vi "ActionVIOnRecompile.vi"(8 "error in":errorcluster, 9 "Timeout (ms)":u32, 10 "Runtime Configurable Section Path":string, 11 "Device Item Ref in":T1 format="%.0x") -> (0 "error out":errorcluster)   [LabVIEW 2020]
uses:
  <vilib>/NI VeriStand/Custom Device API/Custom Device Item Ref.ctl
  <vilib>/NI VeriStand/Custom Device API/Custom Device Channel Type.ctl
  <vilib>/NI VeriStand/Custom Device API/Data Access Type.ctl
  <vilib>/NI VeriStand/Execution/CustomDevice/NI VeriStand - Send Custom Device Message (Byte Array).vi
  <vilib>/NI VeriStand/Custom Device API/Custom Device API.lvlib
  <vilib>/NI VeriStand/Execution/CustomDevice/NI_VS Custom Device ExecutionAPI.lvlib
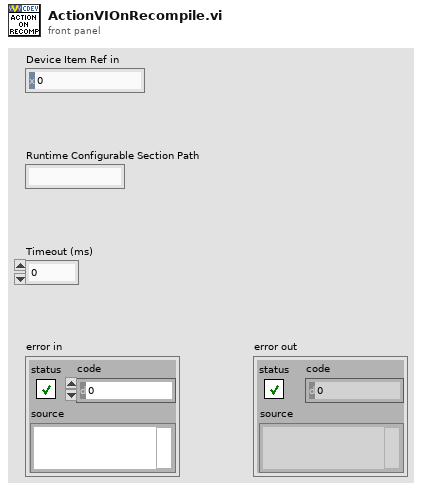
[diagram p1: front panel]
types:
  T1 = typedef "Custom Device API.lvlib/Custom Device Item Ref.ctl" = u64
  T2 = typedef "Custom Device API.lvlib/Custom Device Channel Type.ctl" = enum16{"Input", "Output"}
  T3 = typedef "Custom Device API.lvlib/Data Access Type.ctl" = enum16{"Read", "Write"}
  T4 = typedef "Custom Device API.lvlib/Custom Device Item Info.ctl" = cluster{"Name":string, "Is Channel":bool, "GUID":string, "Is Waveform":bool}
  T5 = typedef "NI_VS Custom Device ExecutionAPI.lvlib/Custom Device Ref.ctl" = refnum<k24>
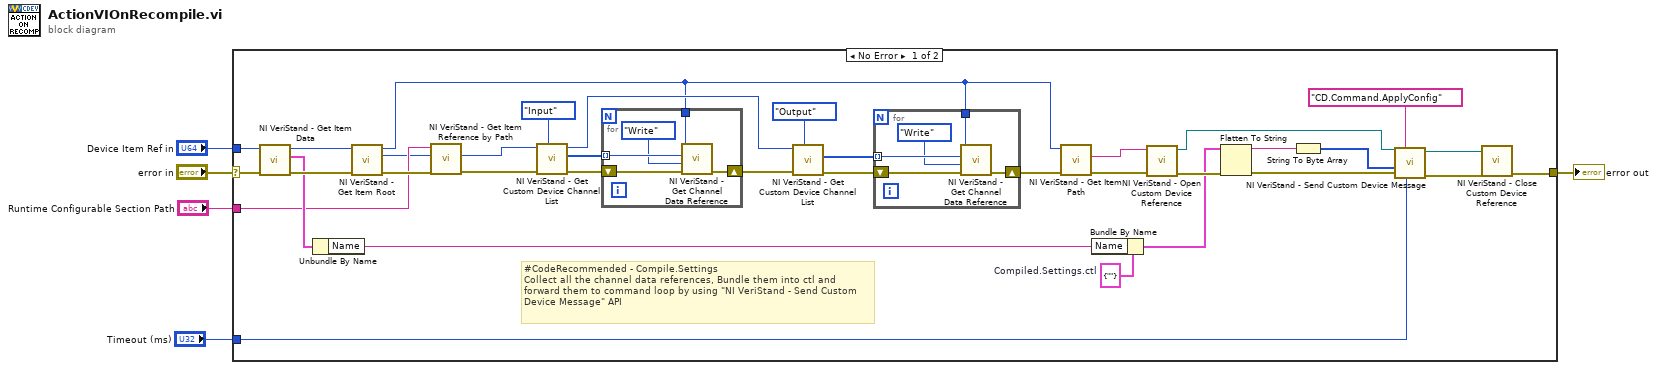
[diagram p0: block diagram]
diagram:
  n1 = case shown="No Error" "error in" {
    selector: "error in" -> [w40 w51]
    tunnel: [w29 w51] -> w4
    tunnel: "Device Item Ref in" -> [w27 _]
    tunnel: "Runtime Configurable Section Path" -> [w22 _]
    tunnel: "Timeout (ms)" -> [w9 _]
    frame No Error {
      w24 = cluster{"Name":string} {"Name"=""}  # Compiled.Settings.ctl
      # "#CodeRecommended - Compile.Settings\nCollect all the channel data references, Bundle them into ctl and forward them to command loop by using \"NI VeriStand - Send Custom Device Message\" API"
      n2 = call <vilib>:"NI VeriStand - Get Item Data.vi"("error in (no error)"=w40, "Item Ref in"=w27) -> ("error out"=w39:errorcluster, "Item Info"=w26:T4, "Item Ref out"=w23:T1)  [unwired: 6 in, 1 out]
      n3 = Unbundle By Name(w26) -> ("Name"=w25:string)
      n4 = call <vilib>:"NI VeriStand - Get Item Root.vi"("error in (no error)"=w39, "Item Ref in"=w23) -> ("error out"=w38:errorcluster, "Root Ref out"=w21:T1, "Item Ref out"=w6:T1)  [unwired: 6 in, 1 out]
      n5 = call <vilib>:"NI VeriStand - Get Item Reference by Path.vi"("error in (no error)"=w38, "Root Ref"=w21, "Item Path in"=w22) -> ("error out"=w37:errorcluster, "Item Ref"=w16:T1)  [unwired: 5 in, 2 out]
      n6 = call <vilib>:"NI VeriStand - Get Custom Device Channel List.vi"("Channel Type"=Custom_Device_Channel_Type."Input", "error in (no error)"=w37, "Device Ref in"=w16) -> ("error out"=w36:errorcluster, "Specified Channel Ref List"=w19:T1[], "Device Ref out"=w7:T1)  [unwired: 6 in]
      n7 = for {
        tunnel: w19 -> [w48] mode=indexing
        shift-right: [w49] -> w34
        shift-left: w36 -> [w50]
        tunnel: w6 -> [w46]
        n8 = call <vilib>:"NI VeriStand - Get Channel Data Reference.vi"("error in (no error)"=w50, "Access"=Data_Access_Type."Write", "Channel Ref in"=w48, "Device Ref in"=w46) -> ("error out"=w49:errorcluster)  [unwired: 5 in, 2 out]
      }
      n9 = call <vilib>:"NI VeriStand - Get Custom Device Channel List.vi"("Channel Type"=Custom_Device_Channel_Type."Output", "error in (no error)"=w34, "Device Ref in"=w7) -> ("error out"=w35:errorcluster, "Specified Channel Ref List"=w18:T1[])  [unwired: 6 in, 1 out]
      n10 = for {
        tunnel: w18 -> [w43] mode=indexing
        shift-right: [w44] -> w33
        shift-left: w35 -> [w45]
        tunnel: w6 -> [w41]
        n11 = call <vilib>:"NI VeriStand - Get Channel Data Reference.vi"("error in (no error)"=w45, "Access"=Data_Access_Type."Write", "Channel Ref in"=w43, "Device Ref in"=w41) -> ("error out"=w44:errorcluster)  [unwired: 5 in, 2 out]
      }
      n12 = call <vilib>:"NI VeriStand - Get Item Path.vi"("error in (no error)"=w33, "Item Ref in"=w6) -> ("error out"=w32:errorcluster, "Path"=w15:string)  [unwired: 6 in, 2 out]
      n13 = Bundle By Name(cluster=w24, "Name"=w25) -> (w14:cluster{"Name":string})
      n14 = call <vilib>:"NI VeriStand - Open Custom Device Reference.vi"("error in (no error)"=w32, "Custom Device Path"=w15) -> ("error out"=w31:errorcluster, "Custom Device"=w8:T5)  [unwired: 8 in]
      n15 = Flatten To String(anything=w14, error in (no error)=w31) -> (data string=w13:string, error out=w30:errorcluster)  [unwired: 2 in, 1 out]
      n16 = String To Byte Array(string=w13) -> (unsigned byte array=w12:u8[])
      n17 = call-poly <vilib>:"NI VeriStand - Send Custom Device Message.vi"("Timeout ms (5000)"=w9, "error in (no error)"=w30, "Data"=w12, "Command"="CD.Command.ApplyConfig", "Custom Device in"=w8) -> ("error out"=w28:errorcluster, "Custom Device out"=w10:T5)  [unwired: 4 in, 1 out]
      n18 = call <vilib>:"NI VeriStand - Close Custom Device Reference.vi"("error in (no error)"=w28, "Custom Device"=w10) -> ("error out"=w29:errorcluster)  [unwired: 9 in]
    }
    frame Error {
    }
  }
  "error out" <- w4
